vi "Sequence End Action.vi"(8 "error in (no error)":errorcluster, 10 "Complete":bool, 11 "Tester in":refnum<class "Tester.lvclass">) -> (0 "error out":errorcluster, 3 "Tester out":refnum<class "Tester.lvclass">)   [LabVIEW 2020, in "Tester.lvlib" / "Tester.lvclass"]
uses:
  Tester.lvclass
  Tester.lvclass/Tester.ctl
  Results/Results.lvclass
  Sequence/Sequence.lvclass
  Step/Step.lvclass
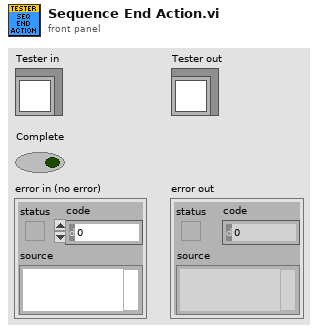
[diagram p1: front panel]
types:
  T1 = typedef "Tester.lvlib/Tester.lvclass/Execution Ref.ctl" = cluster{"Sequence":refnum<class "Sequence.lvclass">, "Step":i32, "Results":refnum<class "Results.lvclass">, "State":T2, "Run Step VI":refnum<vi>, "Abort":bool}
  T2 = typedef "Tester.lvlib/Tester.lvclass/State.ctl" = enum16{"Idle", "In Progress", "Completed"}
  T3 = typedef "Tester.lvlib/Results.lvclass/Result.ctl" = enum16{"No Result", "Pass", "Fail", "Error", "Abort"}
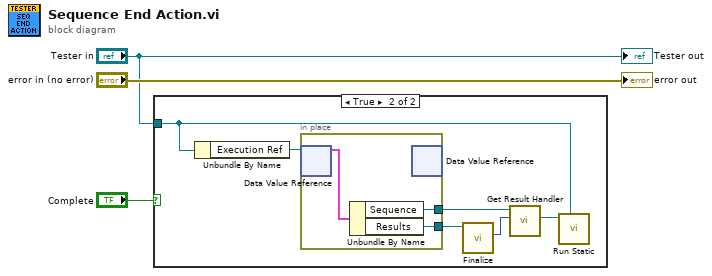
[diagram p0: block diagram]
diagram:
  n1 = case shown="True" "Complete" {
    tunnel: "Tester in" -> [_ w4]
    frame False {
    }
    frame True {
      n2 = Unbundle By Name(w4) -> ("Execution Ref"=w9:refnum<data-value>)
      n3 = in-place {
        in-place-border: [w11] -> w8
        in-place-border: [w10] -> w7
        n4 = in-place-dvr #1(w9) -> (w12:T1)  [unwired: 1 out]
        n5 = Unbundle By Name(w12) -> ("Sequence"=w10:refnum<class "Sequence.lvclass">, "Results"=w11:refnum<class "Results.lvclass">)
        n6 = in-place-dvr #1() -> ()  [unwired: 1 in, 2 out]
      }
      n7 = call "Finalize.vi"("Results in"=w8) -> ("Overall Result"=w6:T3)  [unwired: 8 in, 2 out]
      n8 = call "Get Result Handler.vi"("Result"=w6, "Sequence in"=w7) -> ("Handler"=w5:refnum<class "Step.lvclass">)  [unwired: 7 in, 2 out]
      n9 = call "Run Static.vi"("Tester"=w4, "Step in"=w5) -> ()  [unwired: 8 in, 2 out]
    }
  }
  "error out" <- "error in (no error)"
  "Tester out" <- "Tester in"
